vi "nipkg-createDebianBinaryFile.vi"(8 "error in (no error)":errorcluster, 11 "Package directory":path) -> (0 "error out":errorcluster, 3 "Package directory out":path)   [LabVIEW 2014, in "nipkg-build-system.lvlib"]
uses:
  nipkg-build-system.lvlib
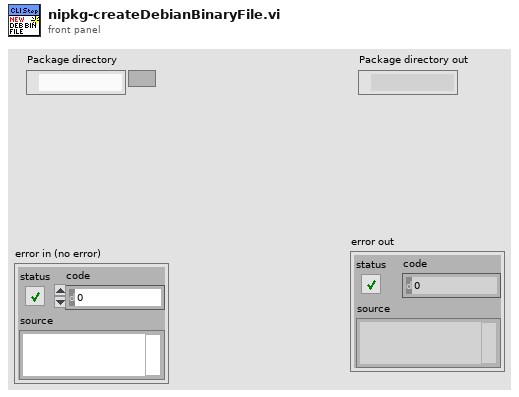
[diagram p1: front panel]
types:
  T1 = enum16{"open", "replace", "create", "open or create", "replace or create", "replace or create with confirmation"}
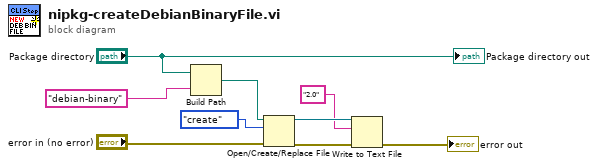
[diagram p0: block diagram]
diagram:
  n1 = Build Path(base path="Package directory", name or relative path="debian-binary") -> (appended path=w7:path)
  n2 = Open/Create/Replace File(file path (use dialog)=w7, error in="error in (no error)", operation (0:open)=T1."create") -> (refnum out=w3:refnum<file>, error out=w4:errorcluster)  [unwired: 3 in, 1 out]
  n3 = Write to Text File(file (use dialog)=w3, text="2.0", error in=w4) -> (error out=→"error out":errorcluster)  [unwired: 1 in, 2 out]
  "Package directory out" <- "Package directory"
